vi "Test Window Position.vi"(11 "Test Case In":refnum<class "Editor Position.lvclass">) -> (0 "error out":errorcluster, 3 "Test Case Out":refnum<class "Editor Position.lvclass">)   [LabVIEW 2021, in "Editor Position.lvclass"]
uses:
  Editor Position.lvclass
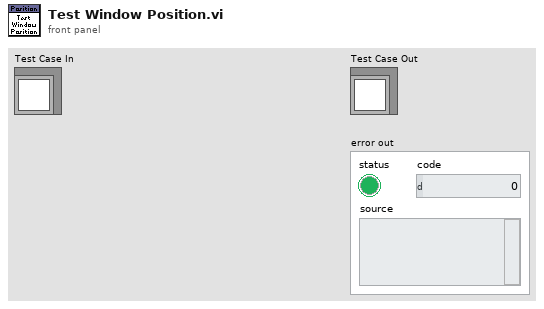
[diagram p1: front panel]
types:
  T1 = enum32{"Invalid", "Standard", "Closed", "Hidden", "Minimized", "Maximized"}
  T2 = typedef "LVRectTypeDef.ctl" = cluster{"Left":i16, "Top":i16, "Right":i16, "Bottom":i16}
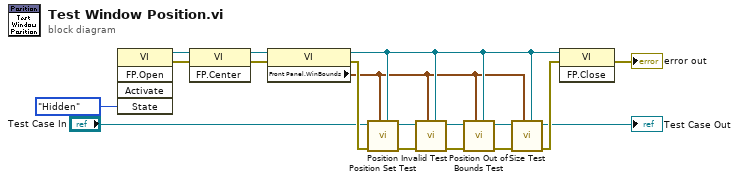
[diagram p0: block diagram]
diagram:
  n1 = invoke class="VI" method="FP.Open"("State"=T1."Hidden") -> (reference out=w9:refnum<vi>, error out=w18:errorcluster)  [unwired: 4 in, 3 out]
  n2 = invoke class="VI" method="FP.Center"(reference=w9, error in=w18) -> (reference out=w8:refnum<vi>, error out=w16:errorcluster)  [unwired: 1 in, 1 out]
  n3 = property class="VI"(reference=w8, error in=w16) -> (reference out=w2:refnum<vi>, error out=w15:errorcluster, "Front Panel.WinBounds"=w1:T2)
  n4 = call "Position Set Test.vi"("VI reference"=w2, "Window Bounds"=w1, "error in"=w15, "Editor Position in"="Test Case In") -> ("error out"=w14:errorcluster, "Editor Position out"=w6:refnum<class "Editor Position.lvclass">)  [unwired: 6 in]
  n5 = call "Position Invalid Test.vi"("VI reference"=w2, "Centered Position"=w1, "error in"=w14, "Editor Position in"=w6) -> ("error out"=w13:errorcluster, "Editor Position out"=w5:refnum<class "Editor Position.lvclass">)  [unwired: 6 in]
  n6 = call "Position Out of Bounds Test.vi"("VI reference"=w2, "Center Bounds"=w1, "error in"=w13, "Editor Position in"=w5) -> ("error out"=w12:errorcluster, "Editor Position out"=w4:refnum<class "Editor Position.lvclass">)  [unwired: 6 in]
  n7 = call "Size Test.vi"("VI reference"=w2, "Center Bounds"=w1, "error in"=w12, "Editor Position in"=w4) -> ("error out"=w11:errorcluster, "Editor Position out"=→"Test Case Out":refnum<class "Editor Position.lvclass">)  [unwired: 6 in]
  n8 = invoke class="VI" method="FP.Close"(reference=w2, error in=w11) -> (error out=→"error out":errorcluster)  [unwired: 1 in, 2 out]
